vi "AcquisitionGlobals.vi"() -> ()   [LabVIEW 2015]
panel:
  out "Abort?":bool
  out "Volumes?":bool
  out "Saving?":bool
  in  "File Save Path":path
  in  "Saving Data?":bool
  out "ImageQueue":refnum<queue>
  out "Acquiring?":bool
  out "Which Laser ON?":bool[](array[boolean])
  in  "Acquisition Mode":string
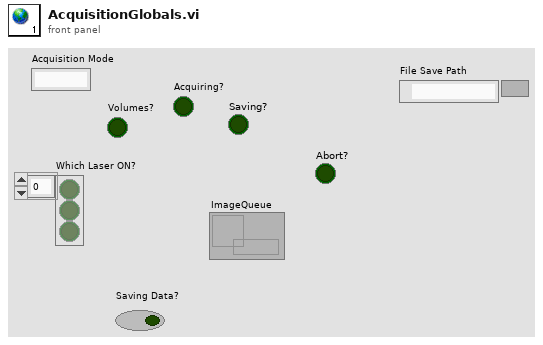
[diagram p1: front panel]
diagram:
